vi "Generate error.vi"(8 "error in (no error)":T1, 10 "info":string, 11 "module":string) -> (0 "error out":T1)   [LabVIEW 2019, in "Shared.lvlib"]
uses:
  Shared.lvlib
  Error event data.ctl
  Comm GV.vi
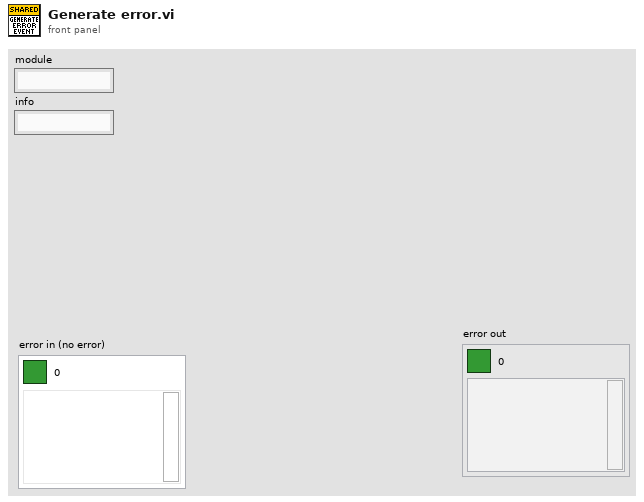
[diagram p1: front panel]
types:
  T1 = cluster{"Boolean Round":bool, "code":i32, "source":string}
  T2 = typedef "Shared.lvlib/Error event data.ctl" = cluster{"module":string, "info":string, "error":cluster{"Boolean Round":bool, "code":i32, "source":string}}
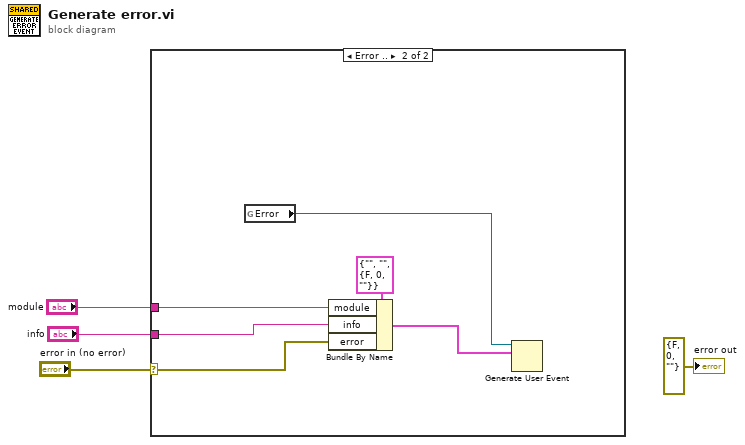
[diagram p0: block diagram]
diagram:
  n1 = case shown="Error .." "error in (no error)" {
    selector: "error in (no error)" -> [_ w7]
    tunnel: "module" -> [_ w6]
    tunnel: "info" -> [_ w5]
    frame No Error {
    }
    frame Error {
      n2 = global read "Comm GV.vi" "Error"() -> (w9:refnum<user-event>)
      n3 = Bundle By Name(cluster=T2 {"module"="", "info"="", "error"={"Boolean Round"=FALSE, "code"=0, "source"=""}} ("error msg"), "module"=w6, "info"=w5, "error"=w7) -> (w8:T2)
      n4 = Generate User Event(user event=w9, event data cluster=w8) -> ()  [unwired: 2 in, 2 out]
    }
  }
  "error out" <- T1 {"Boolean Round"=FALSE, "code"=0, "source"=""} ("error out")
